vi "AVS47_write.vi"(5 "File Reference":refnum<file>) -> ()   [LabVIEW 2019]
uses:
  Global/Global Variables/Data_Display_global.vi
  Instrument_Setup.vi
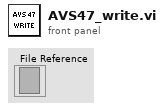
[diagram p1: front panel]
types:
  T1 = typedef "PicowattAVS47-Cluster.ctl" = cluster{"Control Channel (K)":dbl, "AVS CH 5 (Res)":dbl, "AVS CH 6 (Res) ":dbl, "AVS CH 7 (Res) ":dbl, "Control Res.":dbl, "Auto Excitation":bool, "Auto activatet":bool, "AVS Excitation":i16}
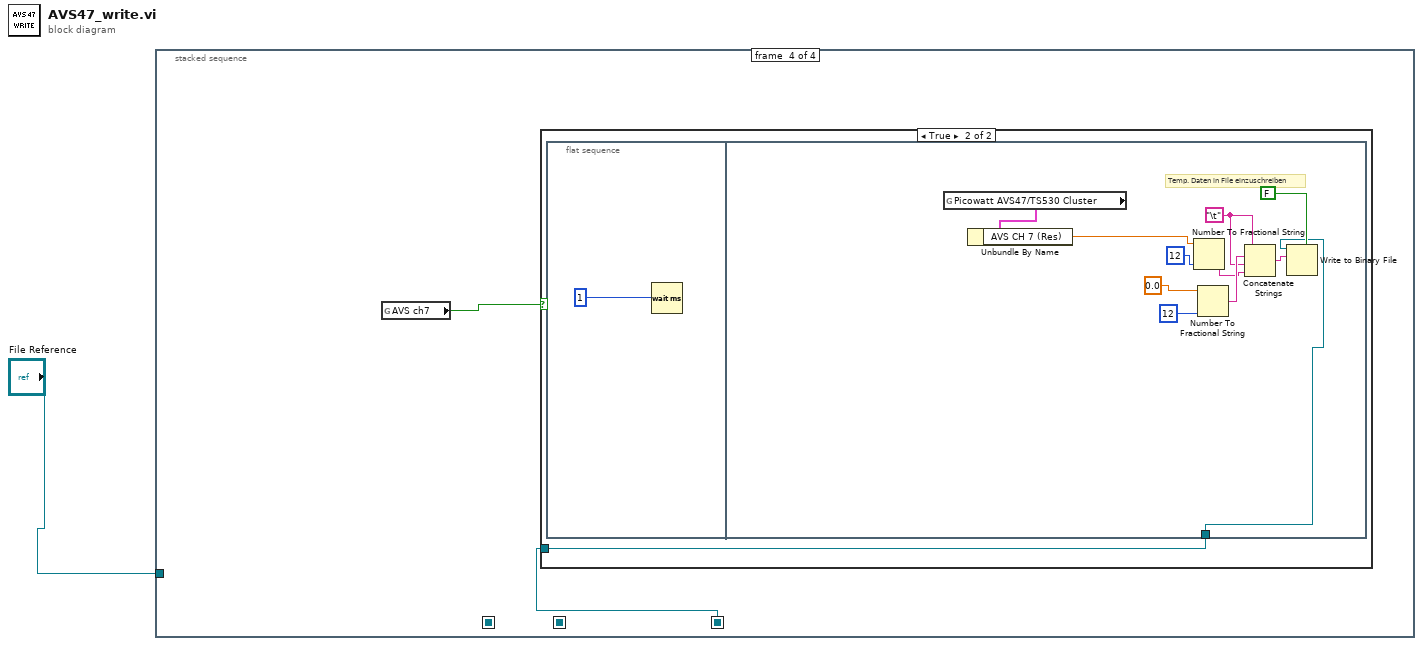
[diagram p0: block diagram]
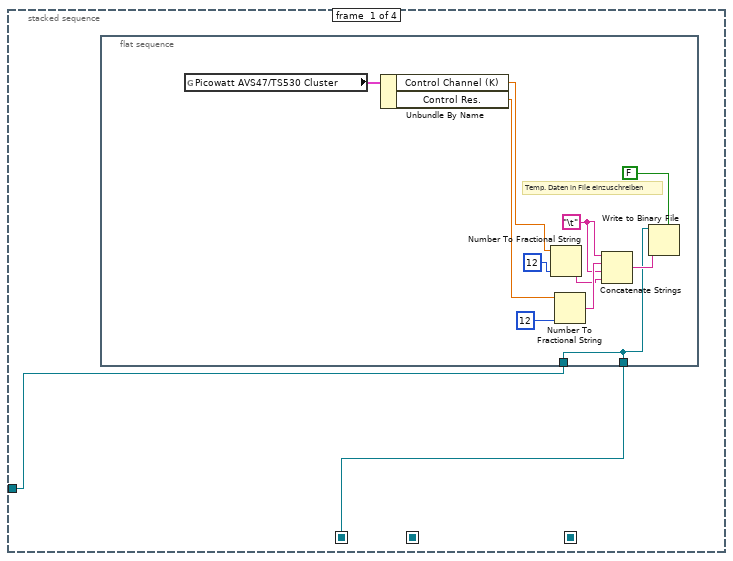
[diagram p2: hidden frame]
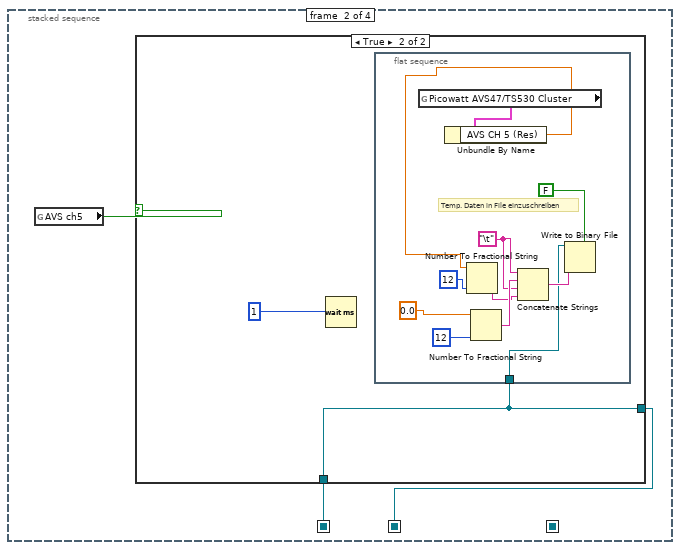
[diagram p3: hidden frame]
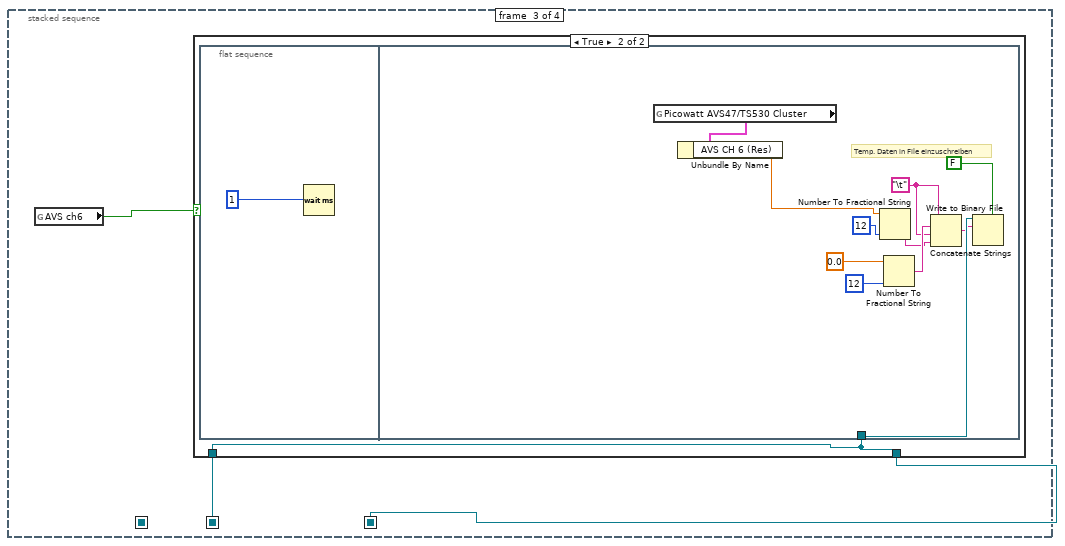
[diagram p5: hidden frame]
diagram:
  n1 = stacked-sequence {
    seq-local: [w2 _ _ _] -> [_ w16 _ _]
    seq-local: [_ w15 _ _] -> [_ _ w33 _]
    seq-local: [_ _ w32 _] -> [_ _ _ w49]
    tunnel: "File Reference" -> [w3 _ _ _]
    frame #0 {
      n2 = flat-sequence {
        tunnel: w3 -> [w4]
        tunnel: [w4] -> w2
        frame #0 {
          w9 = "\t"
          # "Temp. Daten in File einzuschreiben"
          n3 = global read "Data_Display_global.vi" "Picowatt AVS47/TS530 Cluster"() -> (w7:T1)
          n4 = Unbundle By Name(w7) -> ("Control Channel (K)"=w6:dbl, "Control Res."=w5:dbl)
          n5 = Number To Fractional String(number=w6, precision (6)=i16 12) -> (F-format string=w8:string)  [unwired: 2 in]
          n6 = Number To Fractional String(number=w5, precision (6)=i16 12) -> (F-format string=w13:string)  [unwired: 2 in]
          n7 = Concatenate Strings(w9, w13, w9, w8) -> (w14:string)
          n8 = Write to Binary File ("Write File")(file (use dialog)=w4, data=w14, 5:FALSE ("prepend array or string size? (T)")) -> ()  [unwired: 3 in, 3 out]
        }
      }
    }
    frame #1 {
      n9 = global read "Instrument_Setup.vi" "AVS ch5"() -> (w17:bool)
      n10 = case shown="True" w17 {
        tunnel: [w18 w19] -> w15
        tunnel: w16 -> [w18 w19]
        frame False {
        }
        frame True {
          n11 = Wait (ms)(milliseconds to wait=1) -> ()  [unwired: 1 out]
          n12 = flat-sequence {
            tunnel: w19 -> [w24]
            frame #0 {
              w26 = "\t"
              # "Temp. Daten in File einzuschreiben"
              n13 = global read "Data_Display_global.vi" "Picowatt AVS47/TS530 Cluster"() -> (w23:T1)
              n14 = Unbundle By Name(w23) -> ("AVS CH 5 (Res)"=w22:dbl)
              n15 = Number To Fractional String(number=w22, precision (6)=i16 12) -> (F-format string=w25:string)  [unwired: 2 in]
              n16 = Number To Fractional String(number=0.0, precision (6)=i16 12) -> (F-format string=w30:string)  [unwired: 2 in]
              n17 = Concatenate Strings(w26, w30, w26, w25) -> (w31:string)
              n18 = Write to Binary File ("Write File")(file (use dialog)=w24, data=w31, 5:FALSE ("prepend array or string size? (T)")) -> ()  [unwired: 3 in, 3 out]
            }
          }
        }
      }
    }
    frame #2 {
      n19 = global read "Instrument_Setup.vi" "AVS ch6"() -> (w34:bool)
      n20 = case shown="True" w34 {
        tunnel: [w35 w36] -> w32
        tunnel: w33 -> [w35 w36]
        frame False {
        }
        frame True {
          n21 = flat-sequence {
            tunnel: w36 -> [w47]
            frame #0 {
              n22 = Wait (ms)(milliseconds to wait=1) -> ()  [unwired: 1 out]
            }
            frame #1 {
              w43 = "\t"
              # "Temp. Daten in File einzuschreiben"
              n23 = global read "Data_Display_global.vi" "Picowatt AVS47/TS530 Cluster"() -> (w40:T1)
              n24 = Unbundle By Name(w40) -> ("AVS CH 6 (Res)"=w39:dbl)
              n25 = Number To Fractional String(number=w39, precision (6)=i16 12) -> (F-format string=w42:string)  [unwired: 2 in]
              n26 = Number To Fractional String(number=0.0, precision (6)=i16 12) -> (F-format string=w46:string)  [unwired: 2 in]
              n27 = Concatenate Strings(w43, w46, w43, w42) -> (w41:string)
              n28 = Write to Binary File ("Write File")(file (use dialog)=w47, data=w41, 5:FALSE ("prepend array or string size? (T)")) -> ()  [unwired: 3 in, 3 out]
            }
          }
        }
      }
    }
    frame #3 {
      n29 = global read "Instrument_Setup.vi" "AVS ch7"() -> (w50:bool)
      n30 = case shown="True" w50 {
        tunnel: w49 -> [_ w51]
        frame False {
        }
        frame True {
          n31 = flat-sequence {
            tunnel: w51 -> [w56]
            frame #0 {
              n32 = Wait (ms)(milliseconds to wait=1) -> ()  [unwired: 1 out]
            }
            frame #1 {
              w59 = "\t"
              # "Temp. Daten in File einzuschreiben"
              n33 = global read "Data_Display_global.vi" "Picowatt AVS47/TS530 Cluster"() -> (w55:T1)
              n34 = Unbundle By Name(w55) -> ("AVS CH 7 (Res)"=w54:dbl)
              n35 = Number To Fractional String(number=w54, precision (6)=i16 12) -> (F-format string=w58:string)  [unwired: 2 in]
              n36 = Number To Fractional String(number=0.0, precision (6)=i16 12) -> (F-format string=w62:string)  [unwired: 2 in]
              n37 = Concatenate Strings(w59, w62, w59, w58) -> (w57:string)
              n38 = Write to Binary File ("Write File")(file (use dialog)=w56, data=w57, 5:FALSE ("prepend array or string size? (T)")) -> ()  [unwired: 3 in, 3 out]
            }
          }
        }
      }
    }
  }
